vi "Get Read Position.vi"(8 "error in (no error)":errorcluster, 11 "FileStream in":refnum<class "FileStream.lvclass">) -> (0 "error out":errorcluster, 2 "Position":i64, 3 "FileStream out":refnum<class "FileStream.lvclass">)   [LabVIEW 2020, in "Stream.lvlib" / "FileStream.lvclass"]
uses:
  FileStream.lvclass
  FileStream.lvclass/FileStream.ctl
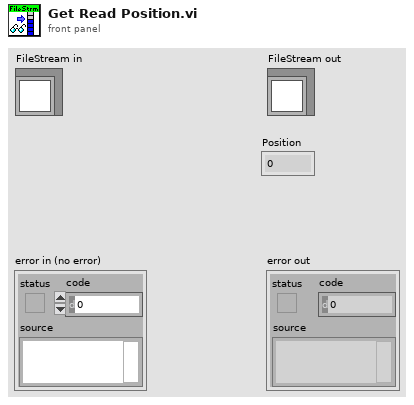
[diagram p1: front panel]
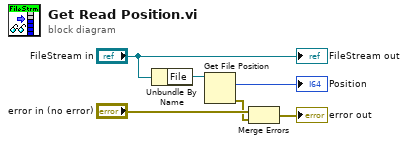
[diagram p0: block diagram]
diagram:
  n1 = Unbundle By Name("FileStream in") -> ("File"=w4:refnum<file>)
  n2 = Get File Position(7:w4) -> (0:w1:errorcluster, 2:→"Position":i64)  [unwired: 1 in, 1 out]
  n3 = Merge Errors("error in (no error)", w1) -> (→"error out":errorcluster)
  "FileStream out" <- "FileStream in"
